vi "New Station Config (Name).vi"(10 "value":map{i32, T1}(c390), 11 "Station Config in":T2) -> (2 "Boolean":bool, 3 "Station Config out":T2)   [LabVIEW 2025, in "Full User Interface.lvlib"]
uses:
  Full User Interface.lvlib
  Station Config.ctl
  Station Info.ctl
  Localization/Section.ctl
  <vilib>/Utility/error.llb/Trim Whitespace One-Sided.vi
  Localization/Localization.lvlib
panel:
  in  "Cancel":bool
  in  "OK":bool
  in  "New Key":string caption="新配方名"
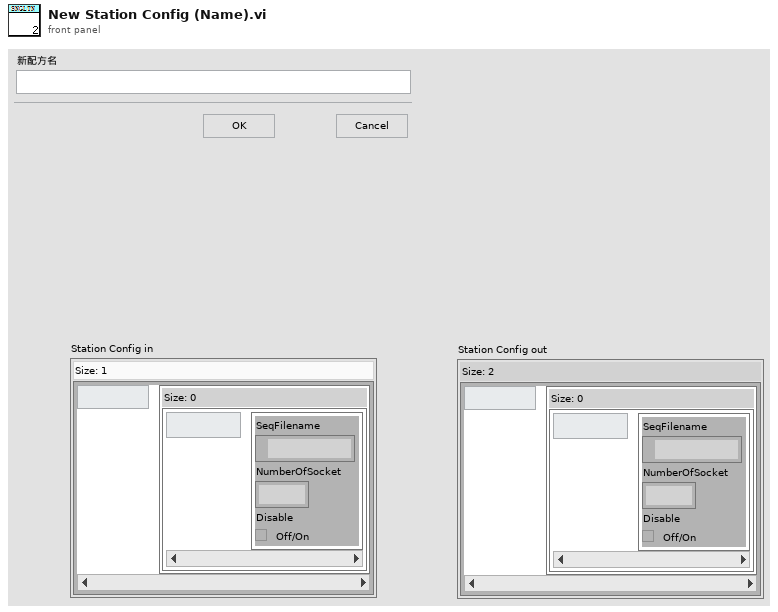
[diagram p1: front panel]
types:
  T1 = typedef "Full User Interface.lvlib/Station Info.ctl" = cluster{"SeqFilename":path, "NumberOfSocket":i32, "Disable":bool}
  T2 = typedef "Full User Interface.lvlib/Station Config.ctl" = map{string, map{i32, T1}}
  T3 = typedef "Localization.lvlib/Section.ctl" = enum16{"Menu", "Title", "Workstation Config"}
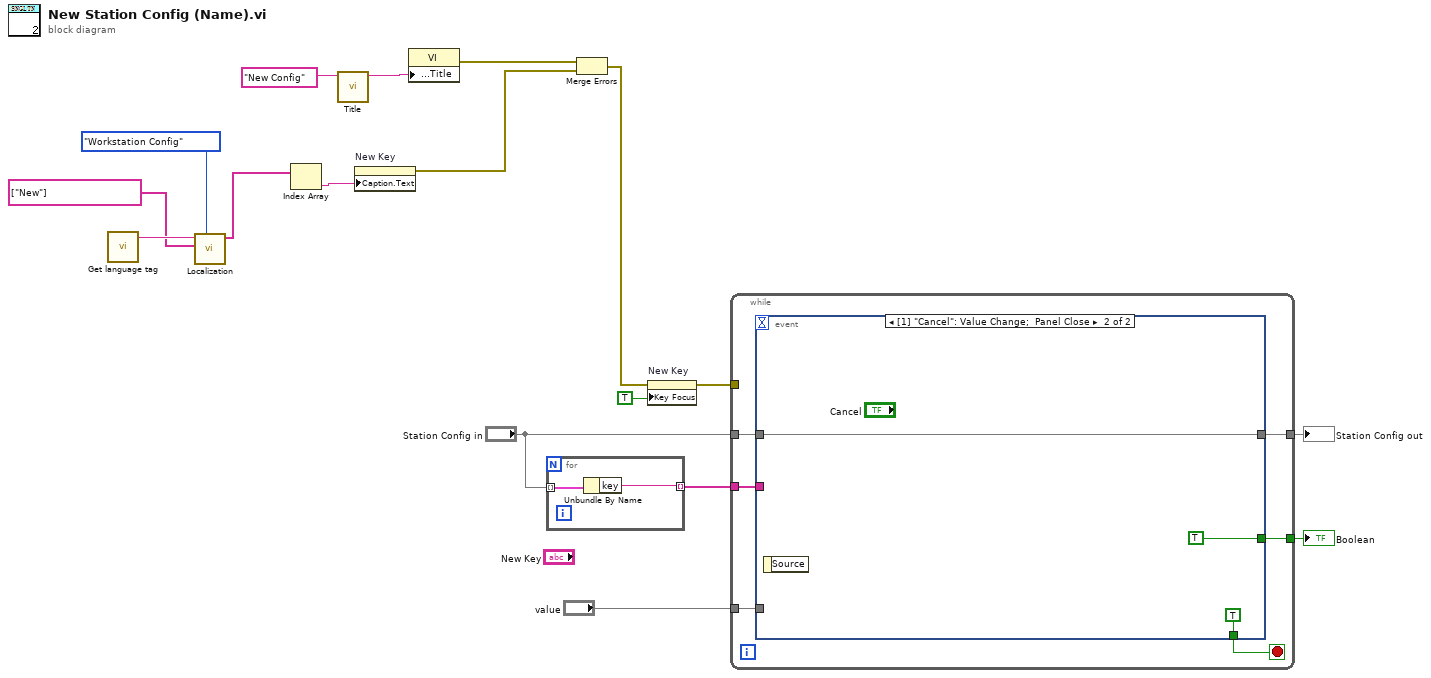
[diagram p0: block diagram]
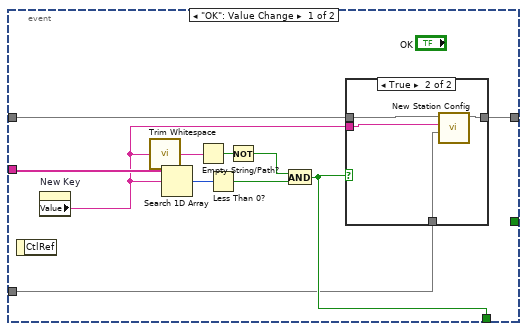
[diagram p2: hidden frame]
diagram:
  n1 = call "Get language tag.vi"() -> ("language tag"=w10:string)  [unwired: 11 in]
  n2 = call "Localization.vi"("section"=Section."Workstation Config", "key"=string[] ["New"], "Language key"=w10) -> ("Value"=w7:string[])  [unwired: 7 in, 1 out]
  n3 = Index Array(array=w7) -> (element=w3:string)  [unwired: 1 in]
  n4 = call "Title.vi"("Front Panel Window:Title"="New Config") -> ("Title"=w11:string)  [unwired: 10 in]
  n5 = property on="New Key" class="Str"("Caption.Text"=w3) -> (error out=w2:errorcluster)  [unwired: 2 in, 1 out]
  n6 = property on="Property Node" class="VI"("Front Panel.Title"=w11) -> (error out=w6:errorcluster)  [unwired: 2 in, 1 out]
  n7 = for {
    tunnel: "Station Config in" -> [w19] mode=indexing
    tunnel: [w18] -> w17 mode=indexing
    n8 = Unbundle By Name(w19) -> ("key"=w18:string)
  }
  n9 = Merge Errors(w6, w2) -> (w5:errorcluster)
  n10 = property on="New Key" class="Str"(error in=w5, "Key Focus"=TRUE) -> (error out=w4:errorcluster)  [unwired: 1 in, 1 out]
  n11 = while {
    tunnel: w17 -> [w25]
    tunnel: "Station Config in" -> [w23]
    tunnel: [w22] -> w15
    tunnel: "value" -> [w21]
    tunnel: w4 -> [_]
    tunnel: [w20] -> w1
    stop <- w24 stop-if-true
    n12 = event shown="[1] \"Cancel\": Value Change;  Panel Close" {
      selector: _ -> [_ _]
      dyn-events: _ -> [_ _]
      timeout: _ -> [_ _]
      tunnel: w25 -> [w36 _]
      tunnel: [w28 TRUE] -> w24
      tunnel: w23 -> [w34 w43]
      tunnel: [w33 w43] -> w22
      tunnel: w21 -> [w26 _]
      tunnel: [_ TRUE] -> w20
      event "OK": Value Change {
        n13 = event-data() -> ()  [unwired: 1 in, 1 out]
        n14 = property on="New Key" class="Str"() -> ("Value"=w31:string)  [unwired: 2 in, 2 out]
        n15 = call <vilib>:"Trim Whitespace.vi"("string"=w31) -> ("trimmed string"=w30:string)  [unwired: 1 in]
        n16 = Search 1D Array(1D array=w36, element=w31) -> (index of element=w35:i32)  [unwired: 1 in]
        n17 = Empty String/Path?(string/path=w30) -> (empty?=w29:bool)
        n18 = Less Than 0?(x=w35) -> (x < 0?=w32:bool)
        n19 = Not(x=w29) -> (.not. x?=w27:bool)
        n20 = And(x=w27, y=w32) -> (x .and. y?=w28:bool)
        n21 = case shown="True" w28 {
          tunnel: w34 -> [w37 w41]
          tunnel: [w37 w40] -> w33
          tunnel: w31 -> [_ w39]
          tunnel: w26 -> [_ w38]
          frame False {
          }
          frame True {
            n22 = call "New Station Config.vi"("value"=w38, "key"=w39, "Station Config in"=w41) -> ("Station Config out"=w40:T2)  [unwired: 8 in]
          }
        }
      }
      event "Cancel": Value Change; Panel Close {
        n23 = event-data() -> ()  [unwired: 1 in, 1 out]
      }
    }
  }
  "Station Config out" <- w15
  "Boolean" <- w1
